vi "Launch Messenger-Commanded Process.vi"(6 "Launch as Slave (F)":bool, 7 "Clone if Reentrant (T)":bool=TRUE, 8 "error in":errorcluster, 11 "VI Refnum":refnum<vi> caption="VI Refnum (will be cloned if reentrant)") -> (0 "error out":errorcluster, 1 "Already Running":bool, 2 "Command Messenger":refnum<class "MGR.lvclass"> caption="Command Messenger to Process", 3 "vi reference":refnum<vi> caption="Process's VI Reference")   [LabVIEW 2011, in "Messenging.lvlib" / "Parallel Process.lvclass"]
doc: "Launchesa VI as a \"Parallel Process\" and returns the command messenger created for that PP (or, if it is already running, just gets the preexisting command messenger)."
uses:
  Parallel Process.lvclass
  Interprocess Messenger/Messenger (Parent)/MGR.lvclass
  Interprocess Messenger/QueueMessenger/QueueMessenger.lvclass
  Interprocess Messenger/TextVarientMessage/MSG.lvclass
  Interprocess Messenger/TextVarientMessage/Write (no data).vi
  Interprocess Messenger/TextVarientMessage/Reply (message).vi
  Interprocess Messenger/TextVarientMessage/Extract Object (static).vi
  Interprocess Messenger/TextVarientMessage/Write VarMessage.vi
  Interprocess Messenger/VarMessage/VarMessage.lvclass
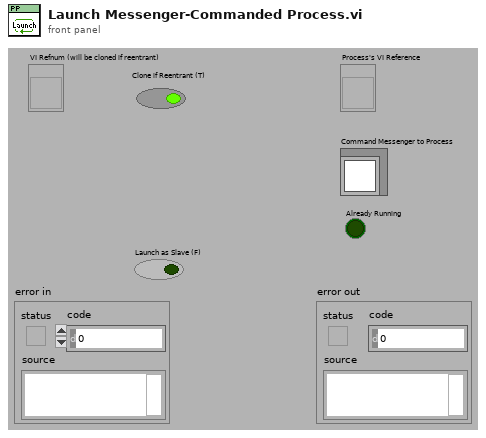
[diagram p1: front panel]
types:
  T1 = enum32{"Bad", "Idle", "Run top level", "Running"}
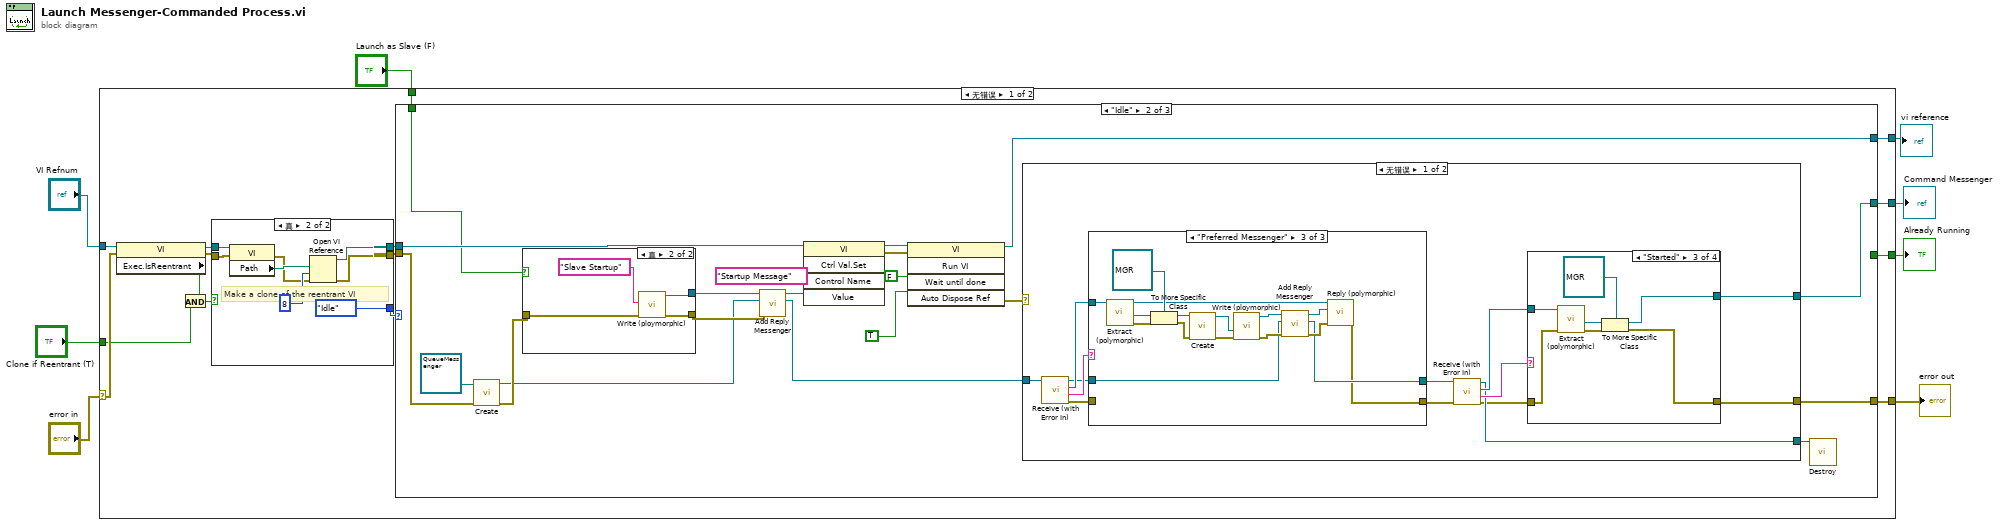
[diagram p0: block diagram]
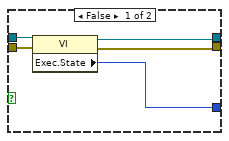
[diagram p2: hidden frame]
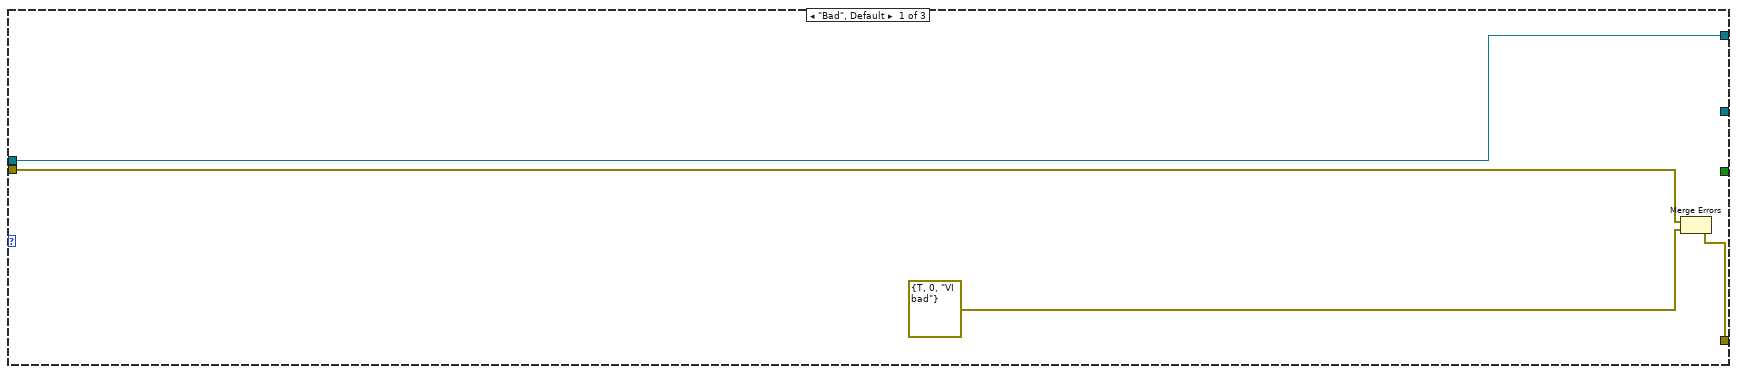
[diagram p3: hidden frame]
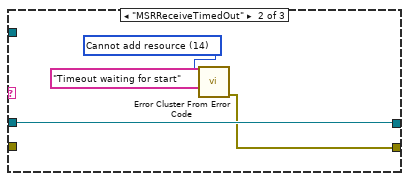
[diagram p5: hidden frame]
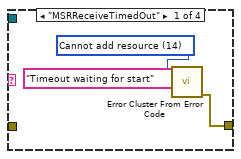
[diagram p6: hidden frame]
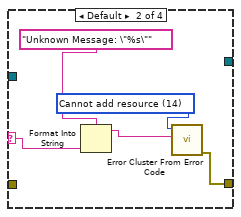
[diagram p7: hidden frame]
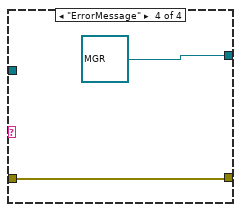
[diagram p8: hidden frame]
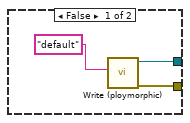
[diagram p10: hidden frame]
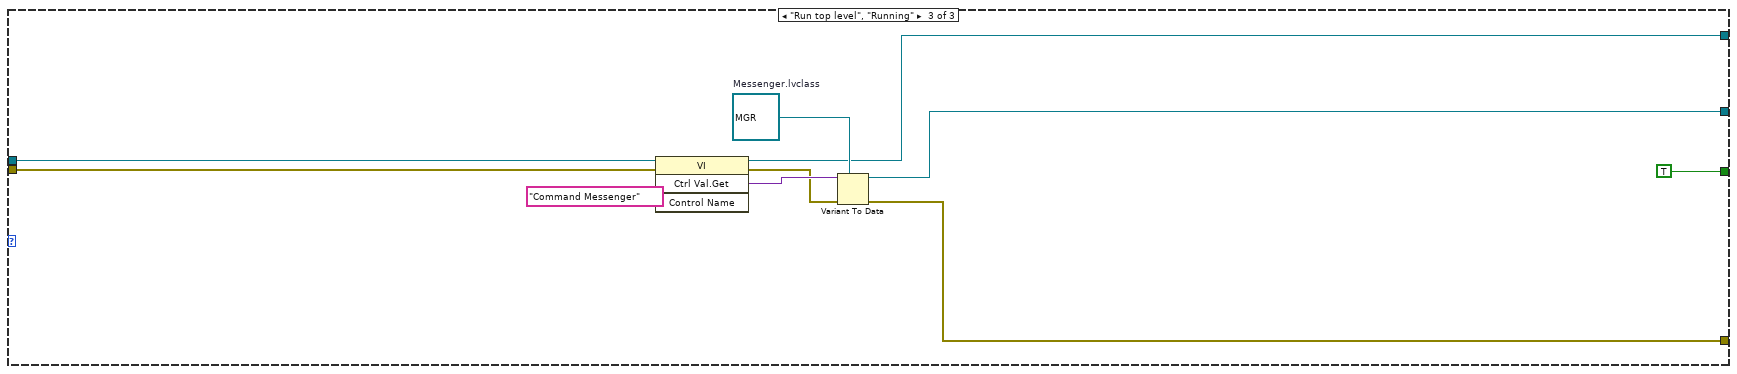
[diagram p11: hidden frame]
diagram:
  n1 = case shown="无错误" "error in" {
    selector: "error in" -> [w13 w133]
    tunnel: [w23 w133] -> w8
    tunnel: [w22 _] -> w7
    tunnel: [w21 w132] -> w6
    tunnel: "VI Refnum" -> [w14 w132]
    tunnel: [w11 _] -> w3
    tunnel: "Launch as Slave (F)" -> [w10 _]
    tunnel: "Clone if Reentrant (T)" -> [w9 _]
    frame No Error {
      n2 = property class="VI"(reference=w14, error in=w13) -> (reference out=w18:refnum<vi>, error out=w19:errorcluster, "Exec.IsReentrant"=w20:bool)
      n3 = And(x=w20, y=w9) -> (x .and. y?=w12:bool)
      n4 = case shown="真" w12 {
        tunnel: w18 -> [w28 w35]
        tunnel: [w26 w30] -> w17
        tunnel: w19 -> [w27 w34]
        tunnel: [w25 w31] -> w16
        tunnel: [w24 T1."Idle" ("Exec.State")] -> w15
        frame False {
          n5 = property class="VI"(reference=w28, error in=w27) -> (reference out=w26:refnum<vi>, error out=w25:errorcluster, "Exec.State"=w24:T1)
        }
        frame True {
          # "Make a clone of the reentrant VI"
          n6 = property class="VI"(reference=w35, error in=w34) -> (error out=w32:errorcluster, "Path"=w33:path)  [unwired: 1 out]
          n7 = Open VI Reference(vi path=w33, options=8, error in (no error)=w32) -> (vi reference=w30:refnum<vi>, error out=w31:errorcluster)  [unwired: 1 in, 2 out]
        }
      }
      n8 = case shown="\"Idle\"" w15 {
        tunnel: [w39 w60 w123] -> w23
        tunnel: [_ w59 w125] -> w22
        tunnel: [w40 w58 w124] -> w21
        tunnel: w17 -> [w40 w53 w127]
        tunnel: w16 -> [w37 w52 w126]
        tunnel: [_ _ TRUE] -> w11
        tunnel: w10 -> [_ w41 _]
        frame "Bad", Default {
          n9 = Merge Errors(w37, errorcluster {"status"=TRUE, "code"=0, "source"="VI bad"} ("error out")) -> (w39:errorcluster)
        }
        frame "Idle" {
          n10 = call-dynamic "Create.vi"("error in (no error)"=w52, "QueueMessenger in"=refnum<class "QueueMessenger.lvclass"> refnum ("QueueMessenger.lvclass")) -> ("error out"=w46:errorcluster, "QueueMessenger out"=w44:refnum<class "QueueMessenger.lvclass">)  [unwired: 8 out]
          n11 = case shown="真" w41 {
            tunnel: [w117 w119] -> w51
            tunnel: w46 -> [_ w120]
            tunnel: [w115 w118] -> w45
            frame False {
              n12 = call-poly "Write (ploymorphic).vi"("Label"="default" ("Text")) -> ("error out"=w115:errorcluster, "Message"=w117:refnum<class "MSG.lvclass">)  [unwired: 1 in, 8 out]
            }
            frame True {
              n13 = call-poly "Write (ploymorphic).vi"("error in (no error)"=w120, "Label"="Slave Startup" ("Text")) -> ("error out"=w118:errorcluster, "Message"=w119:refnum<class "MSG.lvclass">)  [unwired: 8 out]
            }
          }
          n14 = call "Add Reply Messenger.vi"("error in (no error)"=w45, "Reply to..."=w44, "Message"=w51) -> ("Reply to..."=w49:refnum<class "QueueMessenger.lvclass">, "Message"=w50:refnum<class "MSG.lvclass">)  [unwired: 7 out]
          n15 = invoke class="VI" method="Ctrl Val.Set"(reference=w53, "Control Name"="Startup Message", "Value"=w50) -> (reference out=w56:refnum<vi>, error out=w57:errorcluster)  [unwired: 2 in, 3 out]
          n16 = invoke class="VI" method="Run VI"(reference=w56, error in=w57, "Wait until done"=FALSE ("Wait Until Done"), "Auto Dispose Ref"=TRUE ("Auto Dispose Ref (T)")) -> (reference out=w58:refnum<vi>, error out=w43:errorcluster)  [unwired: 1 in, 3 out]
          n17 = case shown="无错误" w43 {
            selector: w43 -> [_ w113]
            tunnel: [w67 w113] -> w60
            tunnel: [w73 _] -> w59
            tunnel: w49 -> [w72 w114]
            tunnel: [w62 w114] -> w42
            frame No Error {
              n18 = call-dynamic "Receive (with Error In).vi"("MGR in"=w72) -> ("error out"=w68:errorcluster, "Label"=w71:string, "Message"=w70:refnum<class "MSG.lvclass">, "MGR out"=w69:refnum<class "QueueMessenger.lvclass">)  [unwired: 2 in, 5 out]
              n19 = case shown="\"Preferred Messenger\"" w71 {
                tunnel: w70 -> [_ _ w90]
                tunnel: w69 -> [w74 w79 w82]
                tunnel: [w74 w79 w81] -> w66
                tunnel: w68 -> [w75 _ _]
                tunnel: [w75 w76 w80] -> w65
                frame "OK", Default {
                }
                frame "MSRReceiveTimedOut" {
                  w77 = 14 items=["No error", "Argument error", "Memory is full", "Out of zone", "End of file", "File already open", "Generic file I/O error", "File not found", "File permission error", "Disk is full", "Duplicate path", "Too many files open", "System feature not enabled", "Resource file not found", "Cannot add resource", "Resource not found", "Image not found", "Image memory error", "Pen does not exist", "Config type invalid", "Config token not found", "Config parse error", "Config memory error", "Bad external code format", "Bad external code offset", "External code not present", "Null window", "Destroy window error", "Null menu", "Print aborted", "Bad print record", "Print driver error", "Windows error during printing", "Memory error during printing", "Print dialog error", "Generic print error", "Invalid device refnum", "Device not found", "Device parameter error", "Device unit error", "Cannot open device", "Device call aborted", "Generic error", "Cancelled by user", "Object ID too low", "Object ID too high", "Object not in heap", "Unknown heap", "Unknown object (invalid DefProc)", "Unknown object (DefProc not in table)", "Message out of range", "Invalid (null) method", "Unknown message", "Manager call not supported", "Bad address", "Network operation in progress", "Network operation timed out", "Connection is busy", "Network attribute not supported", "Network error", "Address in use", "System out of memory", "Connection aborted", "Connection refused", "Not connected", "Already connected", "Connection closed", "Initialization error (interapplication manager)", "Bad occurrence", "Wait on unbound occurrence handler", "Occurrence queue overflow", "Datalog type conflict", "Unused", "Unrecognized type (interapplication manager)", "Memory corrupt", "Failed to make temporary DLL", "Old CIN version", "Drag socket not found", "Failed to load drop-object", "Failed to register OLE object", "Failed to release OLE object", "Format specifier type mismatch", "Unknown format specifier", "Too few format specifiers", "Too many format specifiers", "Scan failed", "Newer CIN version", "Error converting to variant", "Runtime menu error", "Password tampered", "Variant attribute not found", "Incompatible variant data type", "Event data is not available", "Event Store is not present", "Occurrence is not found", "Event Queue is not created", "Event info is not available", "Refnum passed is NULL", "Error retrieving Class GUID", "Error retrieving CoClass GUID", "Error retrieving TypeLib GUID.", "Bad built application magic bytes.", "Specific driver is different from the specific driver associated with the Logical Name.", "There is no session opened to the class driver.", "Max Error", "MAX - Error with config objects", "MAX - Error loading configuration", "MAX - Group not supported"]
                  n20 = call <vilib>:"Error Cluster From Error Code.vi"("error message (\"\")"="Timeout waiting for start" ("error message (\"\")"), "error code (0)"=w77) -> ("error out"=w76:errorcluster)  [unwired: 2 in, 5 out]
                }
                frame "Preferred Messenger" {
                  n21 = call-poly "Extract (polymorphic).vi"("ObjMessage in"=w90) -> ("error out"=w95:errorcluster, "Object"=w94:refnum<class>, "ObjMessage out"=w89:refnum<class "MSG.lvclass">)  [unwired: 1 in, 7 out]
                  n22 = To More Specific Class(target class=refnum<class "MGR.lvclass"> refnum ("Messenging.lvlib:MGR.lvclass"), reference=w94, error in=w95) -> (specific class reference=w92:refnum<class "MGR.lvclass">, error out=w91:errorcluster)
                  n23 = call-dynamic "Create.vi"("error in (no error)"=w91, "Messenger in"=w92) -> ("error out"=w87:errorcluster, "Messenger out"=w88:refnum<class "MGR.lvclass">)  [unwired: 8 out]
                  n24 = call-poly "Write (ploymorphic).vi"("error in (no error)"=w87, "Varient"=w88) -> ("error out"=w86:errorcluster, "Message"=w83:refnum<class "VarMessage.lvclass">)  [unwired: 8 out]
                  n25 = call "Add Reply Messenger.vi"("error in (no error)"=w86, "Reply to..."=w82, "Message"=w83) -> ("error out"=w84:errorcluster, "Reply to..."=w81:refnum<class "QueueMessenger.lvclass">, "Message"=w85:refnum<class "VarMessage.lvclass">)  [unwired: 6 out]
                  n26 = call-poly "Reply (polymorphic).vi"("error in (no error)"=w84, "Reply"=w85, "Message to Reply to"=w89) -> ("error out"=w80:errorcluster)  [unwired: 8 out]
                }
              }
              n27 = call-dynamic "Receive (with Error In).vi"("error in (no error)"=w65, "MGR in"=w66) -> ("error out"=w61:errorcluster, "Label"=w63:string, "Message"=w64:refnum<class "MSG.lvclass">, "MGR out"=w62:refnum<class "QueueMessenger.lvclass">)  [unwired: 1 in, 5 out]
              n28 = case shown="\"Started\"" w63 {
                selector: w63 -> [_ w100 _ _]
                tunnel: [_ _ w107 refnum<class "MGR.lvclass"> refnum ("Messenging.lvlib:MGR.lvclass")] -> w73
                tunnel: [w98 w103 w105 w111] -> w67
                tunnel: w64 -> [_ _ w106 _]
                tunnel: w61 -> [_ _ w104 w111]
                frame "MSRReceiveTimedOut" {
                  w97 = 14 items=["No error", "Argument error", "Memory is full", "Out of zone", "End of file", "File already open", "Generic file I/O error", "File not found", "File permission error", "Disk is full", "Duplicate path", "Too many files open", "System feature not enabled", "Resource file not found", "Cannot add resource", "Resource not found", "Image not found", "Image memory error", "Pen does not exist", "Config type invalid", "Config token not found", "Config parse error", "Config memory error", "Bad external code format", "Bad external code offset", "External code not present", "Null window", "Destroy window error", "Null menu", "Print aborted", "Bad print record", "Print driver error", "Windows error during printing", "Memory error during printing", "Print dialog error", "Generic print error", "Invalid device refnum", "Device not found", "Device parameter error", "Device unit error", "Cannot open device", "Device call aborted", "Generic error", "Cancelled by user", "Object ID too low", "Object ID too high", "Object not in heap", "Unknown heap", "Unknown object (invalid DefProc)", "Unknown object (DefProc not in table)", "Message out of range", "Invalid (null) method", "Unknown message", "Manager call not supported", "Bad address", "Network operation in progress", "Network operation timed out", "Connection is busy", "Network attribute not supported", "Network error", "Address in use", "System out of memory", "Connection aborted", "Connection refused", "Not connected", "Already connected", "Connection closed", "Initialization error (interapplication manager)", "Bad occurrence", "Wait on unbound occurrence handler", "Occurrence queue overflow", "Datalog type conflict", "Unused", "Unrecognized type (interapplication manager)", "Memory corrupt", "Failed to make temporary DLL", "Old CIN version", "Drag socket not found", "Failed to load drop-object", "Failed to register OLE object", "Failed to release OLE object", "Format specifier type mismatch", "Unknown format specifier", "Too few format specifiers", "Too many format specifiers", "Scan failed", "Newer CIN version", "Error converting to variant", "Runtime menu error", "Password tampered", "Variant attribute not found", "Incompatible variant data type", "Event data is not available", "Event Store is not present", "Occurrence is not found", "Event Queue is not created", "Event info is not available", "Refnum passed is NULL", "Error retrieving Class GUID", "Error retrieving CoClass GUID", "Error retrieving TypeLib GUID.", "Bad built application magic bytes.", "Specific driver is different from the specific driver associated with the Logical Name.", "There is no session opened to the class driver.", "Max Error", "MAX - Error with config objects", "MAX - Error loading configuration", "MAX - Group not supported"]
                  n29 = call <vilib>:"Error Cluster From Error Code.vi"("error message (\"\")"="Timeout waiting for start" ("error message (\"\")"), "error code (0)"=w97) -> ("error out"=w98:errorcluster)  [unwired: 2 in, 5 out]
                }
                frame Default {
                  w102 = 14 items=["No error", "Argument error", "Memory is full", "Out of zone", "End of file", "File already open", "Generic file I/O error", "File not found", "File permission error", "Disk is full", "Duplicate path", "Too many files open", "System feature not enabled", "Resource file not found", "Cannot add resource", "Resource not found", "Image not found", "Image memory error", "Pen does not exist", "Config type invalid", "Config token not found", "Config parse error", "Config memory error", "Bad external code format", "Bad external code offset", "External code not present", "Null window", "Destroy window error", "Null menu", "Print aborted", "Bad print record", "Print driver error", "Windows error during printing", "Memory error during printing", "Print dialog error", "Generic print error", "Invalid device refnum", "Device not found", "Device parameter error", "Device unit error", "Cannot open device", "Device call aborted", "Generic error", "Cancelled by user", "Object ID too low", "Object ID too high", "Object not in heap", "Unknown heap", "Unknown object (invalid DefProc)", "Unknown object (DefProc not in table)", "Message out of range", "Invalid (null) method", "Unknown message", "Manager call not supported", "Bad address", "Network operation in progress", "Network operation timed out", "Connection is busy", "Network attribute not supported", "Network error", "Address in use", "System out of memory", "Connection aborted", "Connection refused", "Not connected", "Already connected", "Connection closed", "Initialization error (interapplication manager)", "Bad occurrence", "Wait on unbound occurrence handler", "Occurrence queue overflow", "Datalog type conflict", "Unused", "Unrecognized type (interapplication manager)", "Memory corrupt", "Failed to make temporary DLL", "Old CIN version", "Drag socket not found", "Failed to load drop-object", "Failed to register OLE object", "Failed to release OLE object", "Format specifier type mismatch", "Unknown format specifier", "Too few format specifiers", "Too many format specifiers", "Scan failed", "Newer CIN version", "Error converting to variant", "Runtime menu error", "Password tampered", "Variant attribute not found", "Incompatible variant data type", "Event data is not available", "Event Store is not present", "Occurrence is not found", "Event Queue is not created", "Event info is not available", "Refnum passed is NULL", "Error retrieving Class GUID", "Error retrieving CoClass GUID", "Error retrieving TypeLib GUID.", "Bad built application magic bytes.", "Specific driver is different from the specific driver associated with the Logical Name.", "There is no session opened to the class driver.", "Max Error", "MAX - Error with config objects", "MAX - Error loading configuration", "MAX - Group not supported"]
                  n30 = Format Into String(format string="Unknown Message: \"%s\"" ("error message (\"\")"), w100) -> (resulting string=w99:string)  [unwired: 2 in, 1 out]
                  n31 = call <vilib>:"Error Cluster From Error Code.vi"("error message (\"\")"=w99, "error code (0)"=w102) -> ("error out"=w103:errorcluster)  [unwired: 2 in, 5 out]
                }
                frame "Started" {
                  n32 = call-poly "Extract (polymorphic).vi"("error in (no error)"=w104, "ObjMessage in"=w106) -> ("error out"=w110:errorcluster, "Object"=w109:refnum<class>)  [unwired: 8 out]
                  n33 = To More Specific Class(target class=refnum<class "MGR.lvclass"> refnum ("Messenging.lvlib:MGR.lvclass"), reference=w109, error in=w110) -> (specific class reference=w107:refnum<class "MGR.lvclass">, error out=w105:errorcluster)
                }
                frame "ErrorMessage" {
                }
              }
            }
            frame Error {
            }
          }
          n34 = call-dynamic "Destroy.vi"("QueueMessenger in"=w42) -> ()  [unwired: 1 in, 10 out]
        }
        frame "Run top level", "Running" {
          w128 = refnum<class "MGR.lvclass"> refnum  # Messenger.lvclass
          n35 = invoke class="VI" method="Ctrl Val.Get"(reference=w127, error in=w126, "Control Name"="Command Messenger") -> (reference out=w124:refnum<vi>, error out=w129:errorcluster, "Get Control Value Variant"=w130:variant)  [unwired: 1 in, 1 out]
          n36 = Variant To Data(error in=w129, type=w128, Variant=w130) -> (data=w125:refnum<class "MGR.lvclass">, error out=w123:errorcluster)
        }
      }
    }
    frame Error {
    }
  }
  "error out" <- w8
  "Command Messenger" <- w7
  "vi reference" <- w6
  "Already Running" <- w3
